vi "FindValidCycles.vi"(2 "C (Fix)":u32, 3 "B (+x)":u32, 4 "A (Fix)":u16) -> (0 "D":u32, 1 "B Out":u32)   [LabVIEW 2011]
panel:
  out "Primes 3":i32[](array[numeric])
  out "Primes 2":i32[](array[numeric])
  out "Primes":i32[](array[numeric])
  # "x"
  # "x"
  # "="
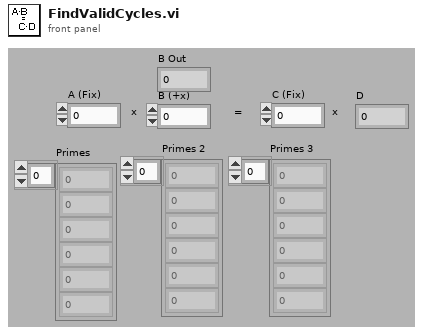
[diagram p1: front panel]
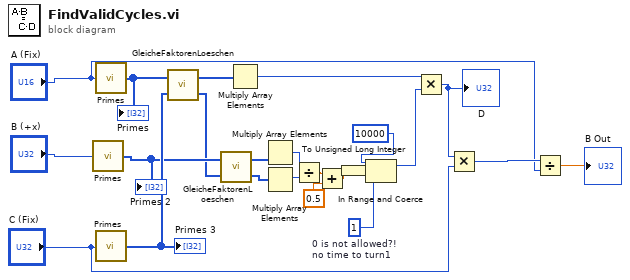
[diagram p0: block diagram]
diagram:
  w5 = u32 1  # 0 is not allowed?! no time to turn1
  n1 = call "Primes.vi"("Numeric"="B (+x)") -> ("Primes"=w20:i32[])
  "Primes 2" <- w20
  n2 = call "Primes.vi"("Numeric"="A (Fix)") -> ("Primes"=w21:i32[])
  "Primes" <- w21
  n3 = call "Primes.vi"("Numeric"="C (Fix)") -> ("Primes"=w22:i32[])
  "Primes 3" <- w22
  n4 = call "GleicheFaktorenLoeschen.vi"("Primes B"=w22, "Primes A"=w21) -> ("Primes BOut"=w13:i32[], "Primes AOut"=w19:i32[])
  n5 = call "GleicheFaktorenLoeschen.vi"("Primes B"=w13, "Primes A"=w20) -> ("Primes BOut"=w16:i32[], "Primes AOut"=w18:i32[])
  n6 = Multiply Array Elements(1:w19) -> (0:w17:i32)
  n7 = Multiply Array Elements(1:w18) -> (0:w15:i32)
  n8 = Multiply Array Elements(1:w16) -> (0:w14:i32)
  n9 = Divide(x=w15, y=w14) -> (x/y=w3:dbl)
  n10 = Add(x=w3, y=0.5) -> (x+y=w2:dbl)
  n11 = To Unsigned Long Integer(number=w2) -> (unsigned 32bit integer=w7:u32)
  n12 = In Range and Coerce(upper limit=u32 10000, x=w7, lower limit=w5) -> (coerced(x)=w6:u32)  [unwired: 1 out]
  n13 = Multiply(x=w17, y=w6) -> (x*y=w12:u32)
  "D" <- w12
  n14 = Multiply(x=w12, y="C (Fix)") -> (x*y=w10:u32)
  n15 = Divide(x=w10, y="A (Fix)") -> (x/y=→"B Out":dbl)
